vi "libssh2_sftp_readdir.vi"(7 "buffer maxlen":i32, 8 "error in (no error)":errorcluster, 11 "sftp handle":T2) -> (0 "error out":errorcluster, 1 "attrs":T1, 2 "buffer":string, 3 "no more files":bool)   [LabVIEW 2013, in "libssh2.lvlib"]
doc: "Read directory data from <B>sftp handle</B>."
uses:
  libssh2.lvlib
  SFTP Handle Refnum.ctl
  libssh2_sftp_attributes.ctl
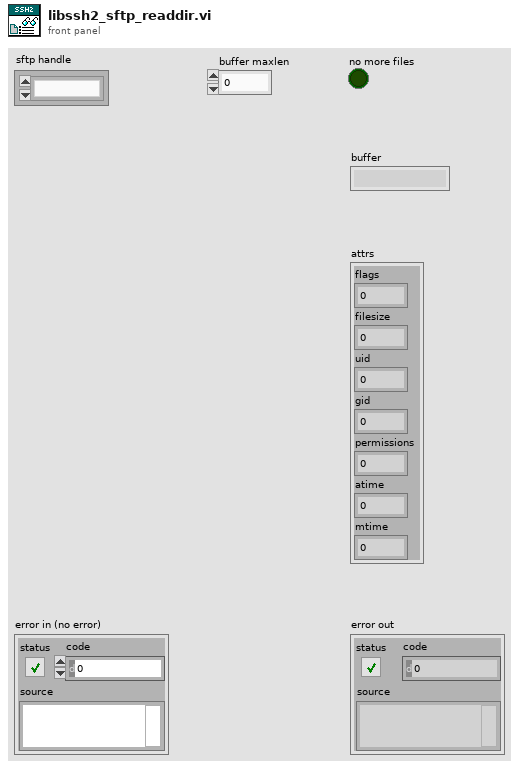
[diagram p1: front panel]
types:
  T1 = typedef "libssh2.lvlib/libssh2_sftp_attributes.ctl" = cluster{"flags":u32, "filesize":u32, "uid":u32, "gid":u32, "permissions":u32, "atime":u32, "mtime":u32}
  T2 = typedef "libssh2.lvlib/SFTP Handle Refnum.ctl" = refnum<k1>
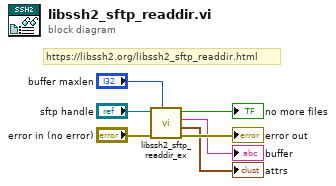
[diagram p0: block diagram]
diagram:
  # "https://libssh2.org/libssh2_sftp_readdir.html"
  n1 = call "libssh2_sftp_readdir_ex.vi"("buffer maxlen"="buffer maxlen", "error in (no error)"="error in (no error)", "sftp handle"="sftp handle") -> ("error out"=→"error out":errorcluster, "attrs"=→"attrs":T1, "buffer"=→"buffer":string, "no more files"=→"no more files":bool)  [unwired: 4 in, 1 out]
